vi "Write Selected.vi"(8 "error in (no error)":errorcluster, 10 "Selected":i16[](array[numeric]), 11 "Editor Handler in":refnum<class "Image Editor Handler.lvclass">) -> (0 "error out":errorcluster, 3 "Editor Handler out":refnum<class "Image Editor Handler.lvclass">)   [LabVIEW 2015, in "LV Image Editor Framework.lvlib" / "Image Editor Handler.lvclass"]
uses:
  Image Editor Handler.lvclass
  Image Editor Handler.lvclass/Image Editor Handler.ctl
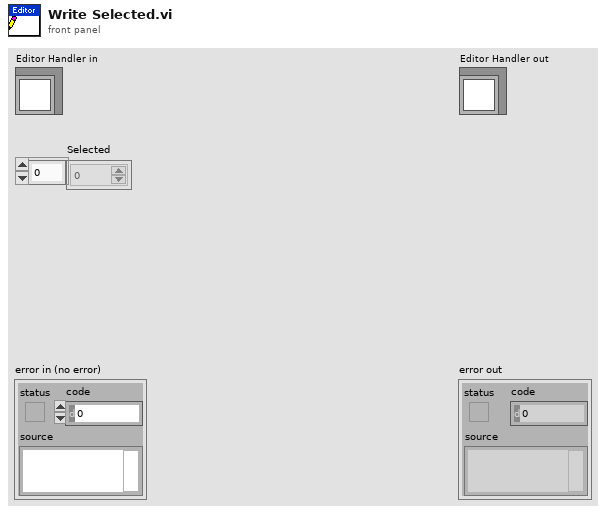
[diagram p1: front panel]
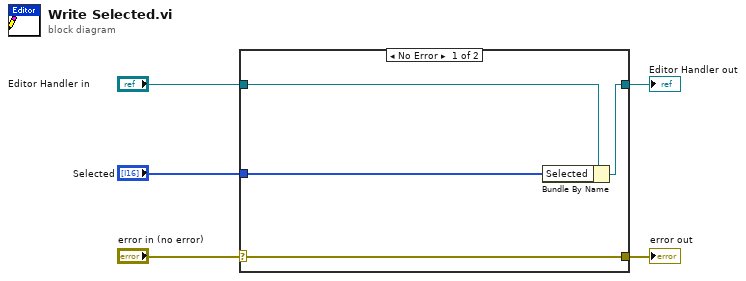
[diagram p0: block diagram]
diagram:
  n1 = case shown="No Error" "error in (no error)" {
    selector: "error in (no error)" -> [w9 w10]
    tunnel: [w9 w10] -> w4
    tunnel: [w7 w11] -> w2
    tunnel: "Editor Handler in" -> [w8 w11]
    tunnel: "Selected" -> [w6 _]
    frame No Error {
      n2 = Bundle By Name(cluster=w8, "Selected"=w6) -> (w7:refnum<class "Image Editor Handler.lvclass">)
    }
    frame Error {
    }
  }
  "error out" <- w4
  "Editor Handler out" <- w2
